vi "Set Port Status.vi"(8 "error in (no error)":errorcluster, 9 "Value":string, 10 "Port":dbl, 11 "object in":refnum<class "Arduino.lvclass">) -> (0 "error out":errorcluster, 3 "object out":refnum<class "Arduino.lvclass">)   [LabVIEW 2020, in "Arduino.lvclass"]
doc: "Set Port Status es el vi donde se escribe el valor del puerto en hexadecimal para que sea recibido por el microcontrolador y pueda encender sus leds correspondientes"
uses:
  Arduino.lvclass
  Arduino.lvclass/Arduino.ctl
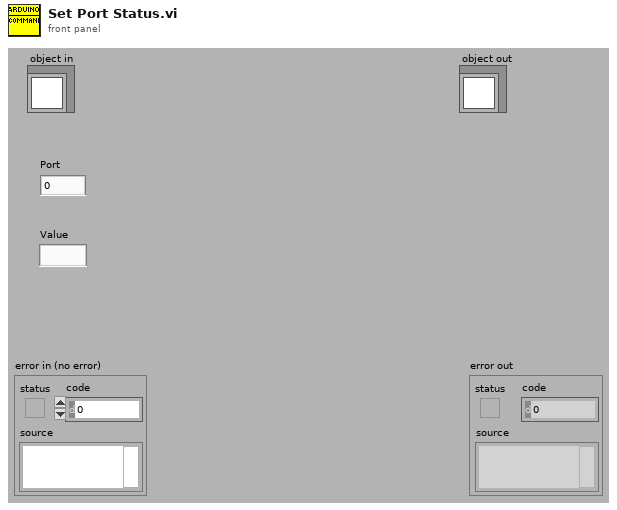
[diagram p1: front panel]
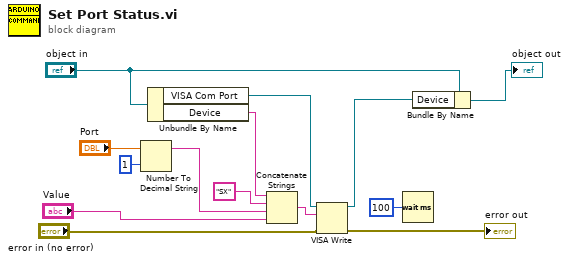
[diagram p0: block diagram]
diagram:
  n1 = Number To Decimal String(number="Port", width (-)=i16 1) -> (decimal integer string=w12:string)
  n2 = Unbundle By Name("object in") -> ("VISA Com Port"=w7:refnum<visa-resource-name>, "Device"=w6:string)
  n3 = Concatenate Strings(w6, "SX" ("string"), w12, "Value") -> (w14:string)
  n4 = VISA Write(VISA resource name=w7, write buffer=w14, error in (no error)="error in (no error)") -> (VISA resource name out=w11:refnum<visa-resource-name>, error out=→"error out":errorcluster)  [unwired: 1 out]
  n5 = Wait (ms)(milliseconds to wait=u32 100) -> ()  [unwired: 1 out]
  n6 = Bundle By Name(cluster="object in", "Device"=w11) -> (→"object out":refnum<class "Arduino.lvclass">)
